vi "HideTheRestCtr.vi"(10 "Array":refnum<vi>[](array[refnum]), 11 "index":i32) -> ()   [LabVIEW 2017]
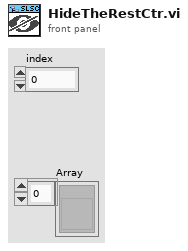
[diagram p1: front panel]
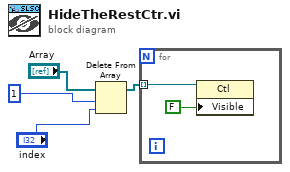
[diagram p0: block diagram]
diagram:
  n1 = Delete From Array(array="Array", length=1, index="index") -> (array with subset deleted=w4:refnum<vi>[])  [unwired: 1 out]
  n2 = for {
    tunnel: w4 -> [w6] mode=indexing
    n3 = property class="Ctl"(reference=w6, "Visible"=FALSE) -> ()  [unwired: 1 in, 2 out]
  }
